vi "Add to Application MUXList.vi"(7 "Replace if found? (F)":bool, 8 "error in (no error)":errorcluster, 9 "Destinations":string[](array[string]), 10 "Source":string, 11 "SLSC Switch in":refnum<class "SLSC Switch.lvclass">) -> (0 "error out":errorcluster, 1 "New Entry?":bool, 3 "SLSC Switch out":refnum<class "SLSC Switch.lvclass">)   [LabVIEW 2016, in "SLSC Switch.lvlib" / "SLSC Switch.lvclass"]
uses:
  SLSC Switch.lvclass
  SLSC Switch.lvclass/SLSC Switch.ctl
  Controls/MuxList Entry.ctl
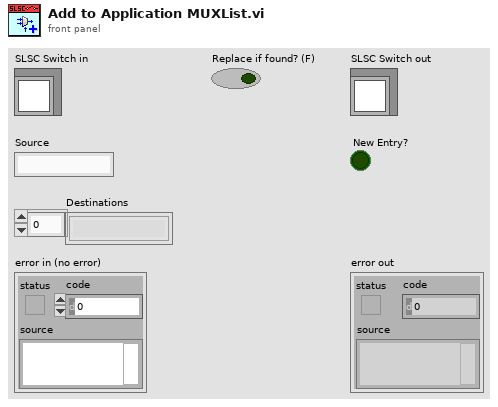
[diagram p1: front panel]
types:
  T1 = typedef "SLSC Switch.lvlib/SLSC Switch.lvclass/MuxList Entry.ctl" = cluster{"Source":string, "Destinations":string[]}
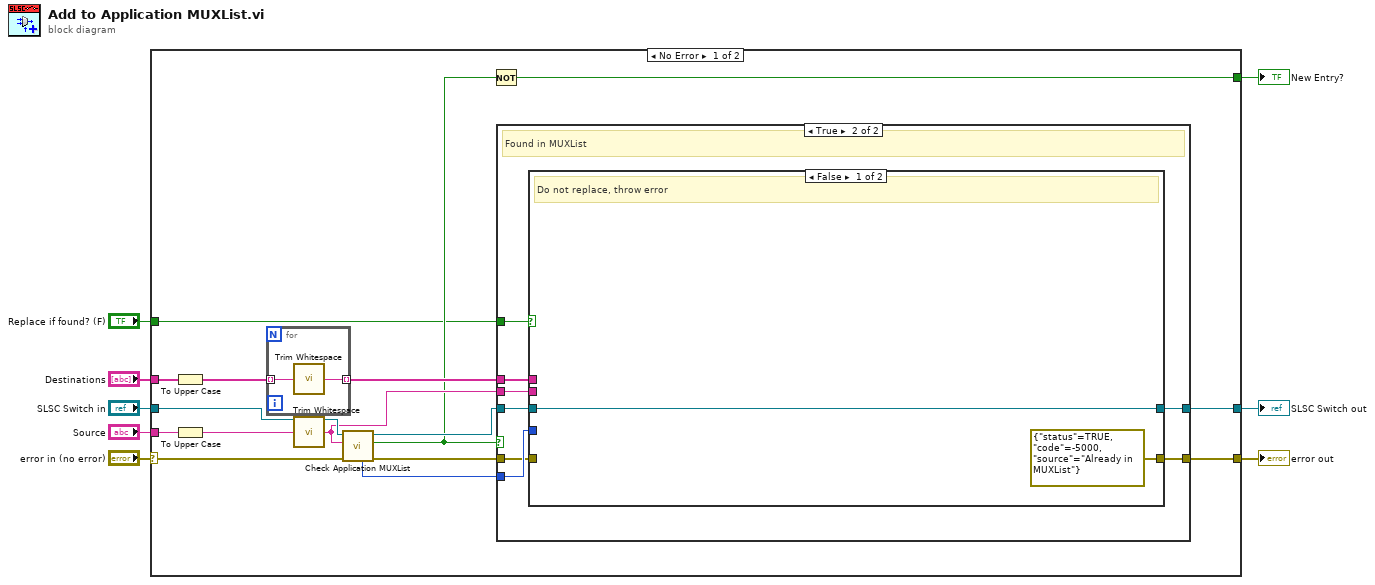
[diagram p0: block diagram]
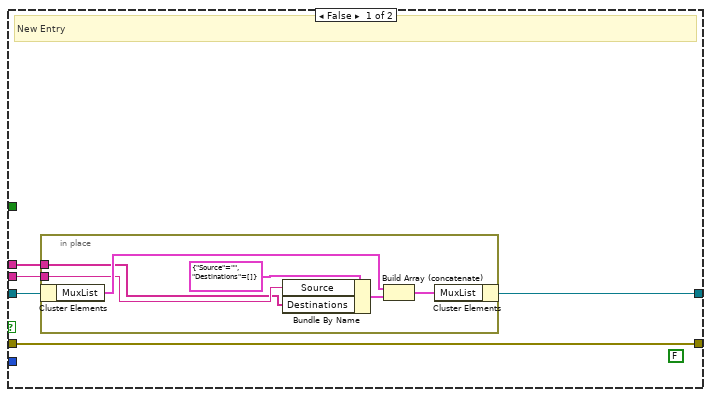
[diagram p2: hidden frame]
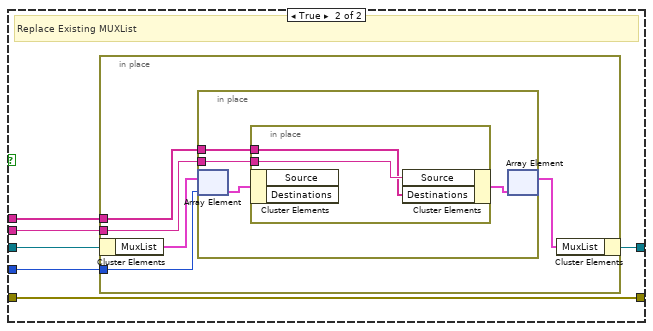
[diagram p3: hidden frame]
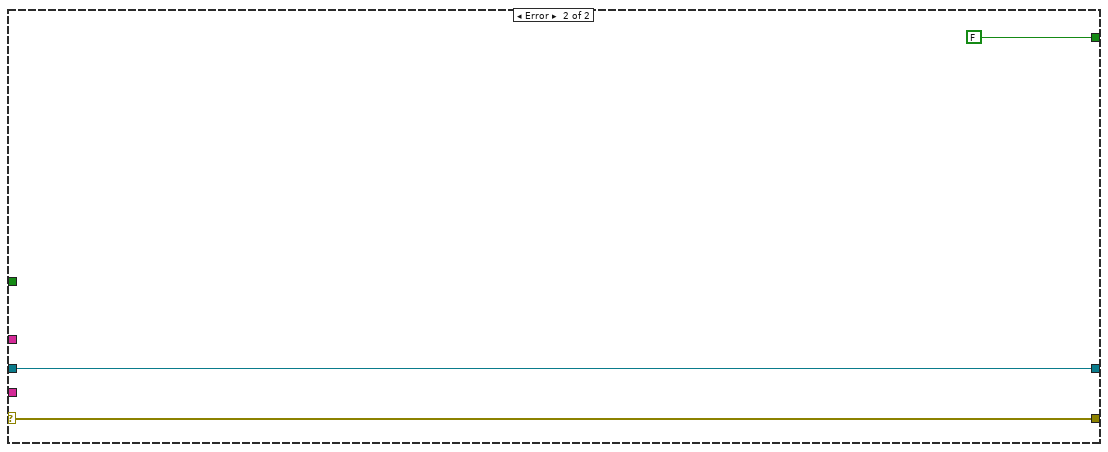
[diagram p4: hidden frame]
diagram:
  n1 = case shown="No Error" "error in (no error)" {
    selector: "error in (no error)" -> [w20 w67]
    tunnel: [w14 w67] -> w7
    tunnel: [w24 w66] -> w5
    tunnel: "SLSC Switch in" -> [w22 w66]
    tunnel: "Source" -> [w12 _]
    tunnel: [w18 FALSE] -> w3
    tunnel: "Destinations" -> [w10 _]
    tunnel: "Replace if found? (F)" -> [w15 _]
    frame No Error {
      n2 = To Upper Case(1:w10) -> (0:w9:string[])
      n3 = To Upper Case(1:w12) -> (0:w11:string)
      n4 = for {
        tunnel: w9 -> [w26] mode=indexing
        tunnel: [w25] -> w23 mode=indexing
        n5 = call <vilib>:"Trim Whitespace.vi"("string"=w26) -> ("trimmed string"=w25:string)  [unwired: 1 in]
      }
      n6 = call <vilib>:"Trim Whitespace.vi"("string"=w11) -> ("trimmed string"=w19:string)  [unwired: 1 in]
      n7 = call "Check Application MUXList.vi"("error in (no error)"=w20, "Source"=w19, "SLSC Switch in"=w22) -> ("error out"=w13:errorcluster, "found?"=w17:bool, "SLSC Switch out"=w21:refnum<class "SLSC Switch.lvclass">, "index"=w16:i32)  [unwired: 4 in, 1 out]
      n8 = Not(x=w17) -> (.not. x?=w18:bool)
      n9 = case shown="True" w17 {
        tunnel: [w31 w40] -> w24
        tunnel: w21 -> [w30 w43]
        tunnel: w19 -> [w29 w42]
        tunnel: w23 -> [w28 w41]
        tunnel: w16 -> [_ w45]
        tunnel: w15 -> [_ w44]
        tunnel: [w27 w39] -> w14
        tunnel: w13 -> [w27 w38]
        frame False {
          (unwired) FALSE
          # "New Entry"
          n10 = in-place {
            in-place-border: w29 -> [w35]
            in-place-border: w28 -> [w34]
            n11 = in-place-cluster #1(w30) -> ("MuxList"=w37:T1[])
            n12 = Bundle By Name(cluster=T1 {"Source"="", "Destinations"=[]} ("Mux"), "Source"=w35, "Destinations"=w34) -> (w33:T1)
            n13 = Build Array (concatenate)(w37, w33) -> (w32:T1[])
            n14 = in-place-cluster #1("MuxList"=w32) -> (w31:refnum<class "SLSC Switch.lvclass">)
          }
        }
        frame True {
          # "Found in MUXList"
          n15 = case shown="False" w44 {
            tunnel: w45 -> [_ w52]
            tunnel: w43 -> [w47 w53]
            tunnel: w42 -> [_ w51]
            tunnel: w41 -> [_ w50]
            tunnel: [w47 w49] -> w40
            tunnel: [errorcluster {"status"=TRUE, "code"=-5000, "source"="Already in MUXList"} ("error out") w48] -> w39
            tunnel: w38 -> [_ w48]
            frame False {
              # "Do not replace, throw error"
            }
            frame True {
              # "Replace Existing MUXList"
              n16 = in-place {
                in-place-border: w52 -> [w57]
                in-place-border: w51 -> [w56]
                in-place-border: w50 -> [w55]
                n17 = in-place-cluster #2(w53) -> ("MuxList"=w58:T1[])
                n18 = in-place {
                  in-place-border: w56 -> [w61]
                  in-place-border: w55 -> [w60]
                  n19 = in-place-array #3(w58, w57) -> (w62:T1)
                  n20 = in-place {
                    in-place-border: w61 -> [w64]
                    in-place-border: w60 -> [w63]
                    n21 = in-place-cluster #4(w62) -> ()  [unwired: 2 out]
                    n22 = in-place-cluster #4("Source"=w64, "Destinations"=w63) -> (w59:T1)
                  }
                  n23 = in-place-array #3(w59) -> (w54:T1[])  [unwired: 1 out]
                }
                n24 = in-place-cluster #2("MuxList"=w54) -> (w49:refnum<class "SLSC Switch.lvclass">)
              }
            }
          }
        }
      }
    }
    frame Error {
    }
  }
  "error out" <- w7
  "SLSC Switch out" <- w5
  "New Entry?" <- w3
